vi "pp2_log_sessionListString.vi"(11 "Session List in":u8[](array[numeric]) min=1 step=1) -> (3 "spreadsheet string":string)   [LabVIEW 2013]
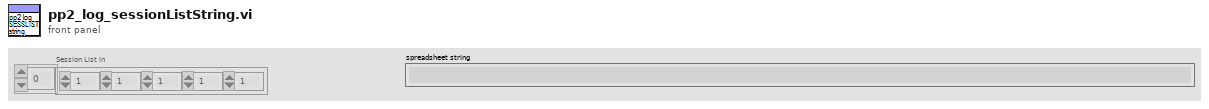
[diagram p1: front panel]
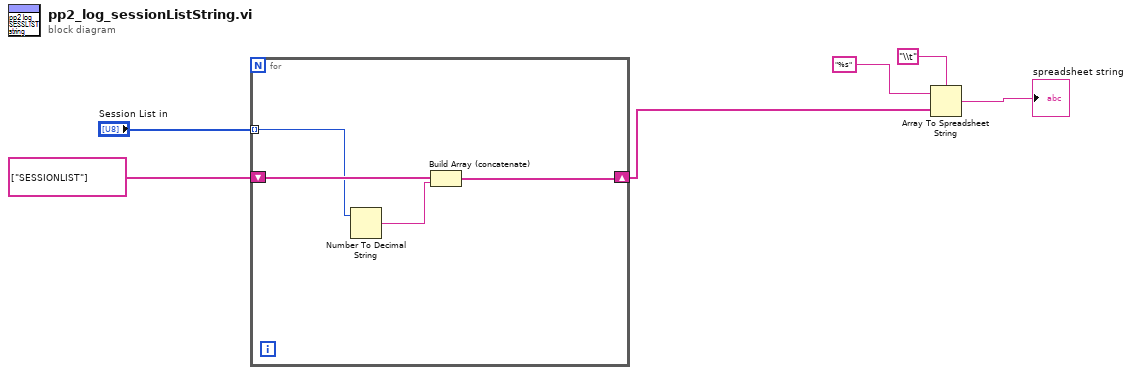
[diagram p0: block diagram]
diagram:
  n1 = for {
    shift-right: [w7] -> w1
    shift-left: string[] ["SESSIONLIST"] -> [w10]
    tunnel: "Session List in" -> [w9] mode=indexing
    n2 = Number To Decimal String(number=w9) -> (decimal integer string=w8:string)  [unwired: 1 in]
    n3 = Build Array (concatenate)(w10, w8) -> (w7:string[])
  }
  n4 = Array To Spreadsheet String(delimiter (Tab)="\\t", array=w1, 3:"%s" ("format string")) -> (spreadsheet string=→"spreadsheet string":string)
